vi "00 Dryer Wilt Call.vi"() -> ()   [LabVIEW 2009]
panel:
  out "Array 2":errorcluster[](array[cluster])
  out "Array":string[](array[string])
  out "Cmds":i32
  in  "error in (no error)":errorcluster
  in  "configuration file path":path=path "C:/work/DryerPerformanceTest.ini"
  in  "data backup command line":string="robocopy \"c:\\Data\" \"XXX\"  "
  in  "update command line":string="robocopy \"XXX\"  \"c:\\Program Files\\GE\\Dryer Performance Test\""
  in  "backup command line":string="robocopy \"c:\\Program Files\\GE\\Dryer Performance Test\"  \"c:\\Program Files\\GE\\backup\""
  out "error out":errorcluster
  in  "command line":string="\"c:\\Program Files\\GE\\Dryer Performance Test\\Dryer Performance Test.exe\""
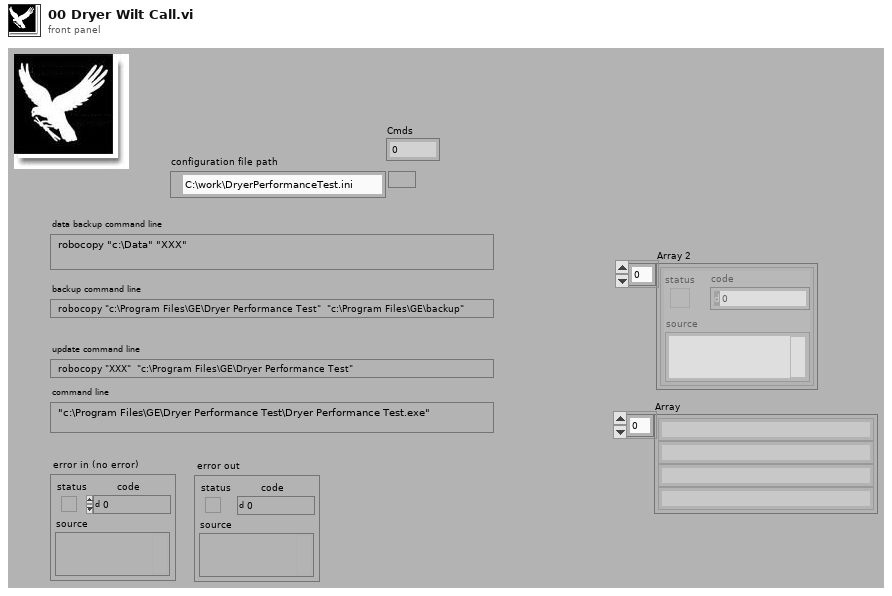
[diagram p1: front panel]
types:
  T1 = typedef "DPT Global Type.ctl" = cluster{"Test Setup":cluster{"3010 resistor":dbl, "Temp Cal":dbl, "Temp Coeff":dbl, "Power On Threshold":dbl, "MA Filter Size":i32, "Weight Offset":dbl, "3011 resistor":dbl, "Gas Enabled":bool, "1020 resistor":dbl}, "Agilent Setup":cluster{"Scale Channel":string, "TC Channels":string, "VDC Discrete Channels":string, "RH Chan":string, "Temp Chan":string, "Tscale Channel":string, "RDB Channel":string, "Gas Temperature":string, "Gas Pressure":string, "Barometric Pressure":string, "Gas Feedback Chan":string}, "Directories":cluster{"Work File Directory":path, "Save File Directory":path, "Library Directory":path, "Data Backup Directory":path}, "Test Information":cluster{"Model:":string, "Temperature:":string, "Engineer:":string, "Technician:":string, "Comments:":string, "Unit:":string, "TR Number:":string, "Test Number:":string, "Test Station:":string, "Empty Dryer Cold Weight:":dbl, "Serial Number:":string, "Build:":string, "Dryer Type":string, "Humidity":string, "Test Title per TR:":string}}
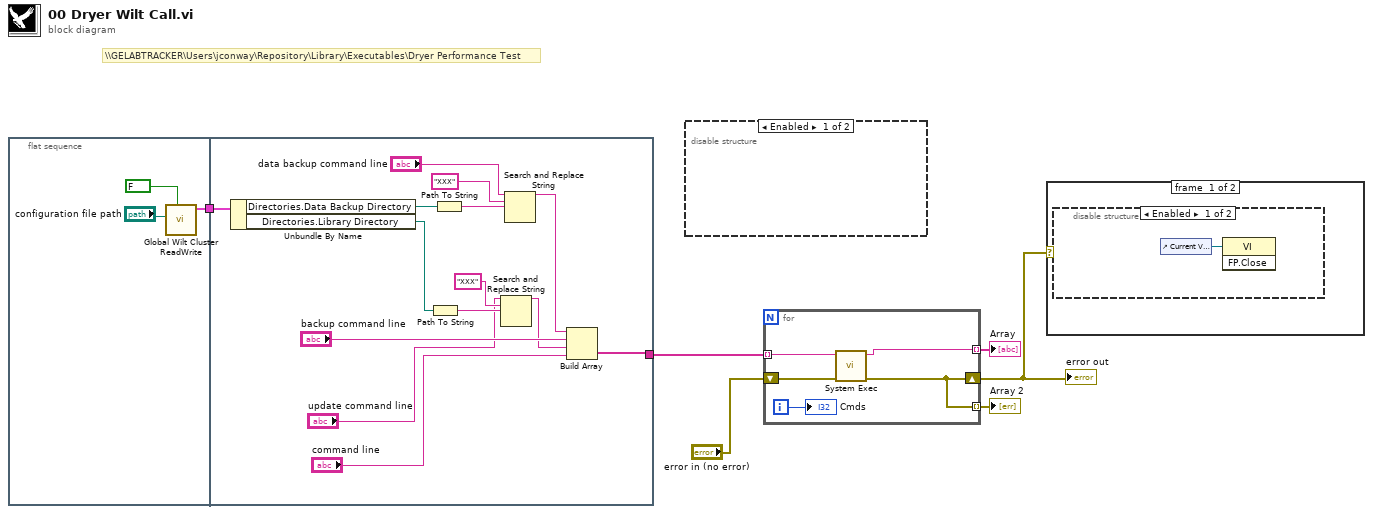
[diagram p0: block diagram]
diagram:
  # "\\\\GELABTRACKER\\Users\\jconway\\Repository\\Library\\Executables\\Dryer Performance Test"
  n1 = flat-sequence {
    tunnel: [w9] -> w5
    tunnel: [w22] -> w6
    tunnel: w5 -> [w19]
    frame #0 {
      n2 = call "Global Wilt Cluster ReadWrite.vi"("Write?"=FALSE, "configuration file path"="configuration file path") -> ("Test Config Out"=w9:T1)  [unwired: 8 in, 1 out]
    }
    frame #1 {
      n3 = Unbundle By Name(w19) -> ("Directories.Data Backup Directory"=w21:path, "Directories.Library Directory"=w13:path)
      n4 = Path To String(path=w13) -> (string=w15:string)
      n5 = Path To String(path=w21) -> (string=w20:string)
      n6 = Search and Replace String(input string="update command line", search string="XXX", replace string=w15) -> (result string=w10:string)  [unwired: 5 in, 3 out]
      n7 = Search and Replace String(input string="data backup command line", search string="XXX", replace string=w20) -> (result string=w16:string)  [unwired: 5 in, 3 out]
      n8 = Build Array(w16, "backup command line", w10, "command line") -> (w22:string[])
    }
  }
  n9 = disable-structure shown="Enabled" {
    frame #0 {
    }
    frame #1 {
    }
  }
  n10 = for {
    tunnel: w6 -> [w28] mode=indexing
    shift-right: [w24] -> w3
    shift-left: "error in (no error)" -> [w27]
    tunnel: [w25] -> w2 mode=indexing
    tunnel: [w24] -> w1 mode=indexing
    i -> [w26]
    n11 = call <vilib>:"System Exec.vi"("error in (no error)"=w27, "command line"=w28) -> ("error out"=w24:errorcluster, "standard output"=w25:string)  [unwired: 6 in, 2 out]
    "Cmds" <- w26
  }
  "error out" <- w3
  "Array" <- w2
  "Array 2" <- w1
  n12 = case shown="No Error" w3 {
    frame #0 {
      n13 = disable-structure shown="Enabled" {
        frame #0 {
          n14 = control-ref of="Current VI Reference"() -> (w29:refnum<vi>)
          n15 = invoke class="VI" method="FP.Close"(reference=w29) -> ()  [unwired: 2 in, 3 out]
        }
        frame #1 {
        }
      }
    }
    frame #1 {
    }
  }
